vi "Create Grid Object.vi"(6 "Label Cluster In":T2, 8 "error in (no error)":errorcluster, 9 "Actual Range In":T1, 10 "3D Plot.lvclass in":refnum<class "3D Plot.lvclass">, 11 "Axis Object In":refnum<vi>) -> (0 "error out":errorcluster, 1 "Actual Range Out":T1, 2 "3D Plot.lvclass out":refnum<class "3D Plot.lvclass">, 3 "Axis Object Out":refnum<vi>, 4 "Label Cluster Out":T2)   [LabVIEW 2020, in "3D Plot.lvclass"]
uses:
  <vilib>/Math Plots/3D Math Plots/3D Plot/3D Plot/3D Plot.lvclass
  <vilib>/Math Plots/3D Math Plots/3D Plot/3D Plot/Typedef/Tick Array Cluster.ctl
  <vilib>/Math Plots/3D Math Plots/3D Plot/3D Plot/Typedef/Tick Array.ctl
  <vilib>/Math Plots/3D Math Plots/3D Plot/3D Plot/Typedef/Range Clusters.ctl
  <vilib>/Math Plots/3D Math Plots/3D Plot/3D Plot/3D Plot.lvclass/3D Plot.ctl
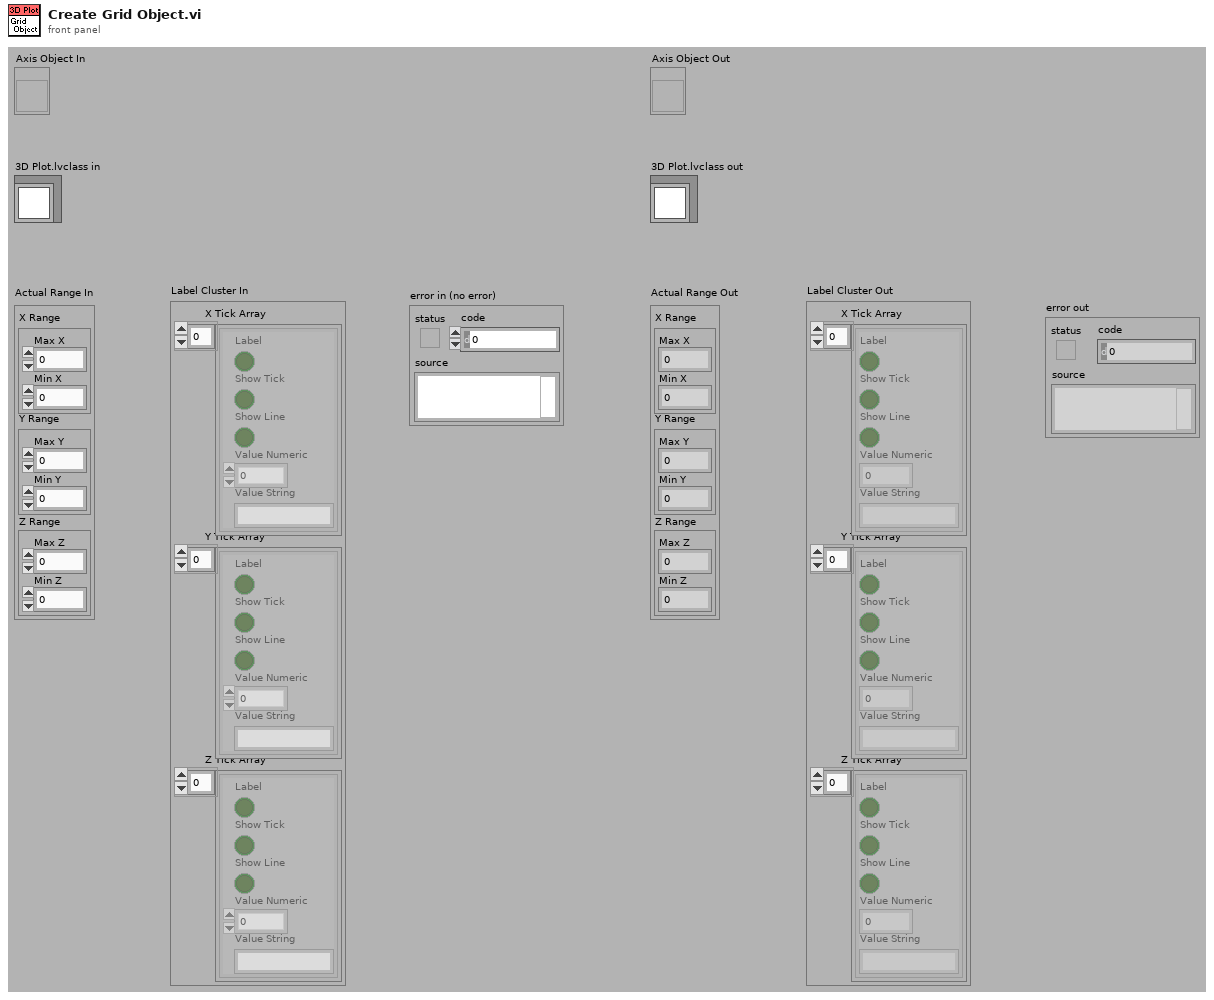
[diagram p1: front panel]
types:
  T1 = typedef "3D Plot.lvclass/Range Clusters.ctl" = cluster{"X Range":cluster{"Max X":sgl, "Min X":sgl}, "Y Range":cluster{"Max Y":sgl, "Min Y":sgl}, "Z Range":cluster{"Max Z":sgl, "Min Z":sgl}}
  T2 = typedef "3D Plot.lvclass/Tick Array Cluster.ctl" = cluster{"X Tick Array":T3, "Y Tick Array":T3, "Z Tick Array":T3}
  T3 = typedef "3D Plot.lvclass/Tick Array.ctl" = cluster{"Label":bool, "Show Tick":bool, "Show Line":bool, "Value Numeric":sgl, "Value String":string}[]
  T4 = cluster{"Draw Grid Plane X-Y":bool, "Draw Grid Plane Y-Z":bool, "Draw Grid Plane X-Z":bool}
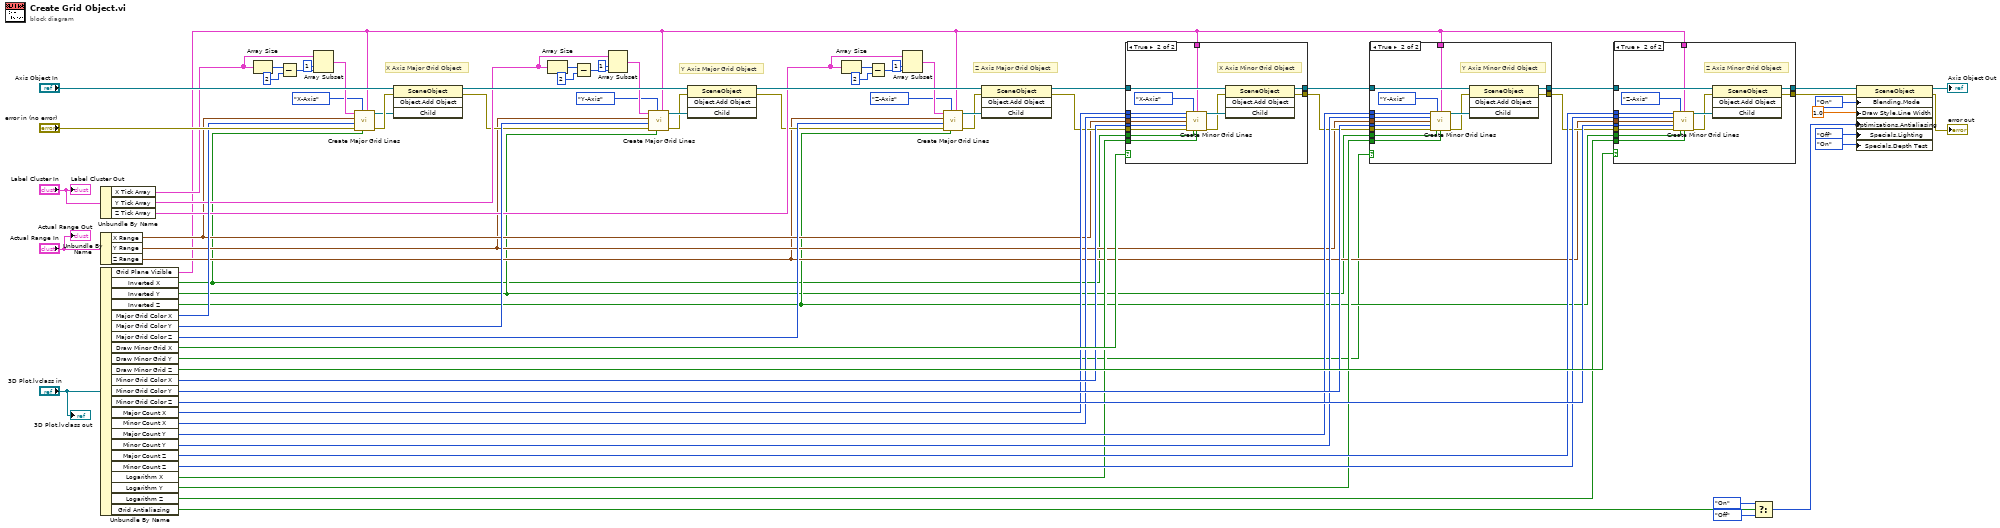
[diagram p0: block diagram]
diagram:
  # "Z Axis Major Grid Object"
  # "Y Axis Major Grid Object"
  # "X Axis Major Grid Object"
  n1 = Unbundle By Name("Label Cluster In") -> ("X Tick Array"=w31:T3, "Y Tick Array"=w67:T3, "Z Tick Array"=w66:T3)
  n2 = Unbundle By Name("Actual Range In") -> ("X Range"=w37:cluster{"Max X":sgl, "Min X":sgl}, "Y Range"=w36:cluster{"Max Y":sgl, "Min Y":sgl}, "Z Range"=w35:cluster{"Max Z":sgl, "Min Z":sgl})
  n3 = Unbundle By Name("3D Plot.lvclass in") -> ("Grid Plane Visible"=w25:T4, "Inverted X"=w32:bool, "Inverted Y"=w33:bool, "Inverted Z"=w34:bool, "Major Grid Color X"=w72:u32, "Major Grid Color Y"=w69:u32, "Major Grid Color Z"=w68:u32, "Draw Minor Grid X"=w57:bool, "Draw Minor Grid Y"=w30:bool, "Draw Minor Grid Z"=w56:bool, "Minor Grid Color X"=w55:u32, "Minor Grid Color Y"=w54:u32, "Minor Grid Color Z"=w53:u32, "Major Count X"=w52:u16, "Minor Count X"=w51:u16, "Major Count Y"=w50:u16, "Minor Count Y"=w49:u16, "Major Count Z"=w48:u16, "Minor Count Z"=w47:u16, "Logarithm X"=w40:bool, "Logarithm Y"=w39:bool, "Logarithm Z"=w38:bool, "Grid Antialiasing"=w28:bool)
  n4 = Array Size(array=w31) -> (size(s)=w20:i32)
  n5 = Subtract(x=w20, y=2) -> (x-y=w22:i32)
  n6 = Array Subset(array=w31, index=1, length=w22) -> (w18:T3)
  n7 = call <vilib>:"Create Major Grid Lines.vi"("Grid Plane Visible"=w25, "Inverted?"=w32, "Axis"=enum16{"X-Axis", "Y-Axis", "Z-Axis"}."X-Axis", "error in (no error)"="error in (no error)", "Grid Color"=w72, "Range"=w37, "Tick Cluster Array"=w18) -> ("error out"=w24:errorcluster, "Grid Object Out"=w23:refnum<vi>)  [unwired: 1 in, 2 out]
  n8 = invoke class="SceneObject" method="Object.Add Object"(reference="Axis Object In", error in=w24, "Child"=w23) -> (reference out=w71:refnum<vi>, error out=w46:errorcluster)  [unwired: 1 in, 2 out]
  n9 = Array Size(array=w67) -> (size(s)=w13:i32)
  n10 = Subtract(x=w13, y=2) -> (x-y=w11:i32)
  n11 = Array Subset(array=w67, index=1, length=w11) -> (w10:T3)
  n12 = call <vilib>:"Create Major Grid Lines.vi"("Grid Plane Visible"=w25, "Inverted?"=w33, "Axis"=enum16{"X-Axis", "Y-Axis", "Z-Axis"}."Y-Axis", "error in (no error)"=w46, "Grid Color"=w69, "Range"=w36, "Tick Cluster Array"=w10) -> ("error out"=w15:errorcluster, "Grid Object Out"=w16:refnum<vi>)  [unwired: 1 in, 2 out]
  n13 = invoke class="SceneObject" method="Object.Add Object"(reference=w71, error in=w15, "Child"=w16) -> (reference out=w70:refnum<vi>, error out=w45:errorcluster)  [unwired: 1 in, 2 out]
  n14 = Array Size(array=w66) -> (size(s)=w4:i32)
  n15 = Subtract(x=w4, y=2) -> (x-y=w6:i32)
  n16 = Array Subset(array=w66, index=1, length=w6) -> (w2:T3)
  n17 = call <vilib>:"Create Major Grid Lines.vi"("Grid Plane Visible"=w25, "Inverted?"=w34, "Axis"=enum16{"X-Axis", "Y-Axis", "Z-Axis"}."Z-Axis", "error in (no error)"=w45, "Grid Color"=w68, "Range"=w35, "Tick Cluster Array"=w2) -> ("error out"=w7:errorcluster, "Grid Object Out"=w8:refnum<vi>)  [unwired: 1 in, 2 out]
  n18 = invoke class="SceneObject" method="Object.Add Object"(reference=w70, error in=w7, "Child"=w8) -> (reference out=w61:refnum<vi>, error out=w44:errorcluster)  [unwired: 1 in, 2 out]
  n19 = case shown="True" w57 {
    tunnel: w55 -> [_ w86]
    tunnel: w61 -> [w81 w95]
    tunnel: [w81 w94] -> w59
    tunnel: w52 -> [_ w92]
    tunnel: w51 -> [_ w91]
    tunnel: w44 -> [w80 w85]
    tunnel: [w80 w93] -> w43
    tunnel: w40 -> [_ w90]
    tunnel: w37 -> [_ w89]
    tunnel: w32 -> [_ w88]
    tunnel: w25 -> [_ w83]
    frame False {
    }
    frame True {
      # "X Axis Minor Grid Object"
      n20 = call <vilib>:"Create Minor Grid Lines.vi"("Major Count"=w92, "Axis"=enum16{"X-Axis", "Y-Axis", "Z-Axis"}."X-Axis", "Grid Plane Visible"=w83, "Minor Count"=w91, "Range"=w89, "Grid Color"=w86, "error in (no error)"=w85, "Inverted?"=w88, "Logarithm?"=w90) -> ("Grid Object Out"=w87:refnum<vi>, "error out"=w84:errorcluster)  [unwired: 1 in, 4 out]
      n21 = invoke class="SceneObject" method="Object.Add Object"(reference=w95, error in=w84, "Child"=w87) -> (reference out=w94:refnum<vi>, error out=w93:errorcluster)  [unwired: 1 in, 2 out]
    }
  }
  n22 = case shown="True" w30 {
    tunnel: w54 -> [_ w104]
    tunnel: w59 -> [w97 w103]
    tunnel: [w97 w102] -> w60
    tunnel: w50 -> [_ w111]
    tunnel: w49 -> [_ w110]
    tunnel: w43 -> [w96 w105]
    tunnel: [w96 w99] -> w42
    tunnel: w39 -> [_ w109]
    tunnel: w36 -> [_ w108]
    tunnel: w33 -> [_ w107]
    tunnel: w25 -> [_ w98]
    frame False {
    }
    frame True {
      # "Y Axis Minor Grid Object"
      n23 = call <vilib>:"Create Minor Grid Lines.vi"("Major Count"=w111, "Axis"=enum16{"X-Axis", "Y-Axis", "Z-Axis"}."Y-Axis", "Grid Plane Visible"=w98, "Minor Count"=w110, "Range"=w108, "Grid Color"=w104, "error in (no error)"=w105, "Inverted?"=w107, "Logarithm?"=w109) -> ("Grid Object Out"=w101:refnum<vi>, "error out"=w100:errorcluster)  [unwired: 1 in, 4 out]
      n24 = invoke class="SceneObject" method="Object.Add Object"(reference=w103, error in=w100, "Child"=w101) -> (reference out=w102:refnum<vi>, error out=w99:errorcluster)  [unwired: 1 in, 2 out]
    }
  }
  n25 = case shown="True" w56 {
    tunnel: w53 -> [_ w121]
    tunnel: [w113 w115] -> w58
    tunnel: w60 -> [w113 w120]
    tunnel: w48 -> [_ w127]
    tunnel: w47 -> [_ w126]
    tunnel: w42 -> [w112 w122]
    tunnel: [w112 w116] -> w41
    tunnel: w38 -> [_ w125]
    tunnel: w35 -> [_ w124]
    tunnel: w34 -> [_ w123]
    tunnel: w25 -> [_ w114]
    frame False {
    }
    frame True {
      # "Z Axis Minor Grid Object"
      n26 = call <vilib>:"Create Minor Grid Lines.vi"("Major Count"=w127, "Axis"=enum16{"X-Axis", "Y-Axis", "Z-Axis"}."Z-Axis", "Grid Plane Visible"=w114, "Minor Count"=w126, "Range"=w124, "Grid Color"=w121, "error in (no error)"=w122, "Inverted?"=w123, "Logarithm?"=w125) -> ("Grid Object Out"=w119:refnum<vi>, "error out"=w118:errorcluster)  [unwired: 1 in, 4 out]
      n27 = invoke class="SceneObject" method="Object.Add Object"(reference=w120, error in=w118, "Child"=w119) -> (reference out=w115:refnum<vi>, error out=w116:errorcluster)  [unwired: 1 in, 2 out]
    }
  }
  n28 = Select(t=enum16{"Inherit Value", "Off", "On"}."On" ("Optimizations:Antialiasing"), s=w28, f=enum16{"Inherit Value", "Off", "On"}."Off" ("Optimizations:Antialiasing")) -> (s? t:f=w26:enum16{"Inherit Value", "Off", "On"})
  n29 = property class="SceneObject"(reference=w58, error in=w41, "Blending.Mode"=enum16{"Inherit Value", "Off", "On"}."On" ("Specials:Lighting"), "Draw Style.Line Width"=sgl 1.0 ("Draw Style:Line Width"), "Optimizations.Antialiasing"=w26, "Specials.Lighting"=enum16{"Inherit Value", "Off", "On"}."Off" ("Blending:Mode"), "Specials.Depth Test"=enum16{"Inherit Value", "Off", "On"}."On" ("Specials:Depth Test")) -> (reference out=→"Axis Object Out":refnum<vi>, error out=→"error out":errorcluster)
  "Label Cluster Out" <- "Label Cluster In"
  "Actual Range Out" <- "Actual Range In"
  "3D Plot.lvclass out" <- "3D Plot.lvclass in"
